vi "Untitled 9.vi"() -> ()   [LabVIEW 2017]
uses:
  JSONtext.lvlib
panel:
  out "error out":errorcluster
  in  "error in (no error)":errorcluster
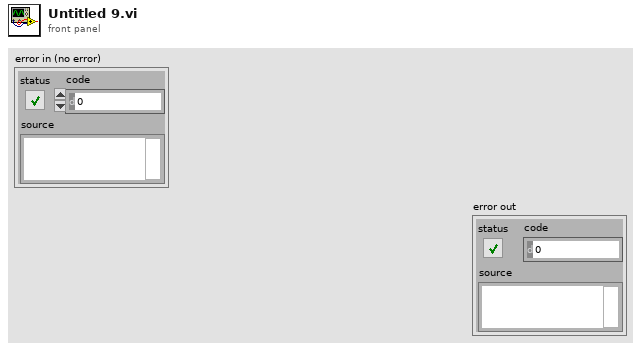
[diagram p1: front panel]
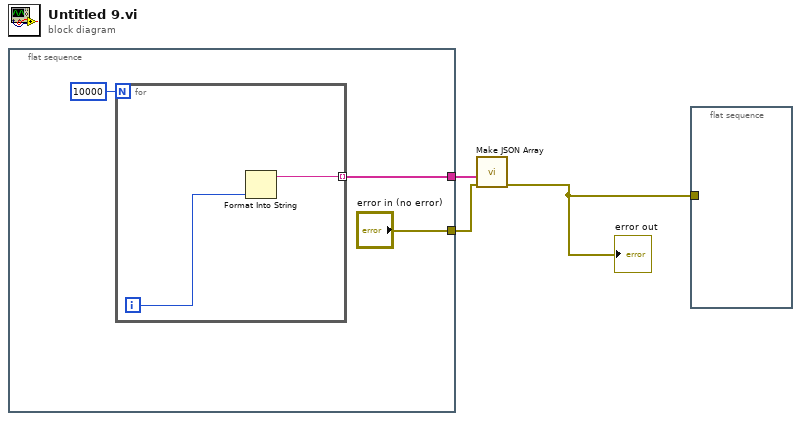
[diagram p0: block diagram]
diagram:
  n1 = flat-sequence {
    tunnel: [w5] -> w3
    tunnel: ["error in (no error)"] -> w2
    frame #0 {
      n2 = for {
        N: 10000 -> [_]
        tunnel: [w7] -> w5 mode=indexing
        i -> [w8]
        n3 = Format Into String(w8) -> (resulting string=w7:string)  [unwired: 3 in, 1 out]
      }
    }
  }
  n4 = call "Make JSON Array.vi"("error in (no error)"=w2, "JSON Elements"=w3) -> ("error out"=w1:errorcluster)  [unwired: 8 in, 1 out]
  "error out" <- w1
  n5 = flat-sequence {
    tunnel: w1 -> [_]
    frame #0 {
    }
  }
